vi "Perform crosstalk measurement.vi"(8 "error in (no error)":errorcluster, 10 "I2S waveforms":waveform(dbl)[](array[waveform]), 11 "measurement configuration":T2={"Full scale range"=2.825, "Channel name"="", "Analog source resource name"="", "Frequency"=0.0, "Amplitude"=0.0, "Protocol capture resource name"="", "Data line"=0, "Interferer channel"=0, "Victim channel"=0, "Sample rate"=44100.0, "Measurement duration"=0.1, "Frame sync edge for channel 0"=1, "Channel count per frame"=2, "Channel length"=32, "Bit depth"=24, "Channel 0 offset"=1, "Endiannes"=0, "Data justification"=0, "Frame length"=64, "Frame sync pulse width"=32, "Bit clock edge sync"=1}) -> (0 "error out":errorcluster, 3 "measurement results":T1)   [LabVIEW 2021, in "Crosstalk_Audio ADC.lvlib"]
uses:
  Crosstalk_Audio ADC.lvlib
  Measurement Configuration.ctl
  Measurement Results.ctl
  <vilib>/addons/_NISVFA/_Shared subVIs/Common/SVL Set dB Reference (N Ch - 1 Ref).vi
  <vilib>/addons/_NISVFA/_Spectrum Processing/SVFA Unit Conversion (Complex) (1 Ch).vi
  <vilib>/addons/_NISVFA/_Shared subVIs/Common/SVL Set dB Reference (1 Ch).vi
  <vilib>/addons/_NISVFA/_Shared subVIs/Common/svc_Log View for Spectrum (1Ch).vi
  <vilib>/addons/_NISVFA/_Spectrum Processing/SVFA Unit Conversion (1 Ch).vi
  <vilib>/addons/_NISVFA/_Shared subVIs/Common/svc_Complex Datatype Defaults.vi
  <vilib>/addons/_NISVFA/_Shared subVIs/Common/SVL Set dB Reference (variant).vi
  <vilib>/addons/_NISVFA/_Shared subVIs/Common/svc_Unwrap Phase.vi
  <vilib>/addons/_NISVFA/_Shared subVIs/Common/svc_Convert Spectrum Array to dB.vi
  <vilib>/addons/_NISVFA/_Shared subVIs/Common/svc_Spectrum Units.vi
  <vilib>/addons/_NISVFA/_Spectrum Processing/subVIs/svfa_Conversion Utility (spectrum info).vi
  <vilib>/addons/_NISVFA/_Shared subVIs/Common/svc_Format Value (DBL).vi
  <vilib>/addons/_NISVFA/_Shared subVIs/Common/svc_Get Weighting Enum and Labels.vi
  <vilib>/addons/_NISVFA/_Shared subVIs/Common/svc_Engineering Units to Unit Label.vi
  <vilib>/addons/_NISVFA/_Shared subVIs/Common/svc_Surround NonAlpha String with Parentheses.vi
  <vilib>/dlg_ctls.llb/Space Constant.vi
  <vilib>/addons/_NISVFA/_Spectrum Processing/subVIs/svfa_Peak to RMS to Peak2Peak.vi
  <vilib>/addons/_NISVFA/_Spectrum Processing/subVIs/svfa_Mag to Mag2.vi
  <vilib>/addons/_NISVFA/_Spectrum Processing/subVIs/svfa_Linear to dB.vi
  <vilib>/addons/_NISVFA/_Spectrum Processing/subVIs/svfa_dBrefA to dBrefB.vi
  <vilib>/addons/_NISVFA/_Spectrum Processing/subVIs/svfa_Spectrum to Spectral Density.vi
  <vilib>/addons/_NISVFA/_Shared subVIs/Common/svc_Unit Label Lexical Class.vi
  <vilib>/addons/_NISVFA/_Shared subVIs/Common/svc_Window Parameters.vi
  <vilib>/addons/_NISVFA/_Shared subVIs/Common/svc_Caller VI Returned in Error Source.vi
  <vilib>/addons/Sound and Vibration/svt_Single Tone Measurements/SVT Crosstalk (Time).vi
  <vilib>/Analysis/4window.llb/window parameters.vi
  <vilib>/Analysis/4window.llb/Window Properties.vi
  <vilib>/Analysis/4window.llb/Window Properties by Name.vi
  <vilib>/addons/Sound and Vibration/svt_Single Tone Measurements/SoundVib_SingleTone.lvlib
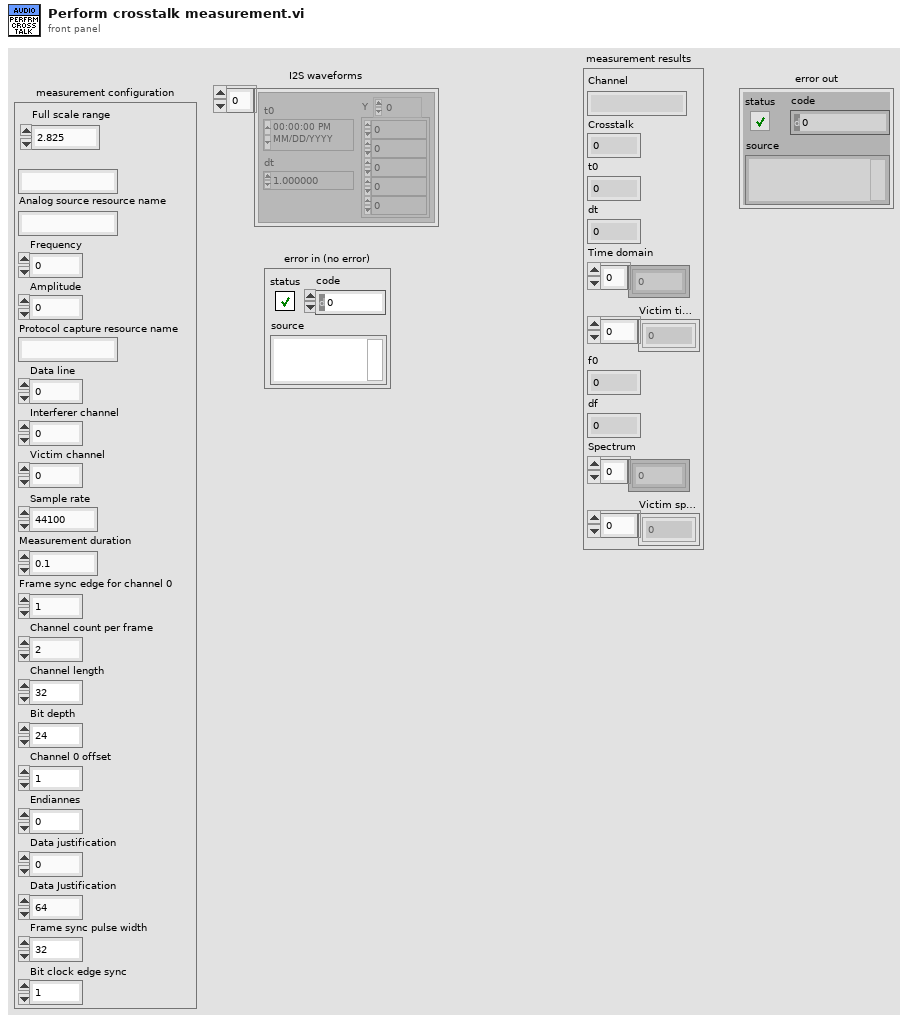
[diagram p1: front panel]
types:
  T1 = typedef "Crosstalk_Audio ADC.lvlib/Measurement Results.ctl" = cluster{"Channel":string, "Crosstalk":dbl, "t0":dbl, "dt":dbl, "Time domain":dbl[], "Victim time domain":dbl[], "f0":dbl, "df":dbl, "Spectrum":dbl[], "Victim spectrum":dbl[]}
  T2 = typedef "Crosstalk_Audio ADC.lvlib/Measurement Configuration.ctl" = cluster{"Full scale range":dbl, "Channel name":string, "Analog source resource name":string, "Frequency":dbl, "Amplitude":dbl, "Protocol capture resource name":string, "Data line":u32, "Interferer channel":u32, "Victim channel":u32, "Sample rate":dbl, "Measurement duration":dbl, "Frame sync edge for channel 0":u32, "Channel count per frame":u32, "Channel length":u32, "Bit depth":u32, "Channel 0 offset":u32, "Endiannes":u32, "Data justification":u32, "Frame length":u32, "Frame sync pulse width":u32, "Bit clock edge sync":u32}
  T3 = enum16{"no change", "spectrum", "spectral density"}
  T4 = cluster{"linear/dB":enum16{"no change", "linear", "dB"}, "dB reference (0: no change)":dbl, "power/magnitude":enum16{"no change", "power", "magnitude"}, "view":enum16{"no change", "rms", "peak", "peak-peak"}}
  T5 = typedef "svc_Spectrum Info.ctl" = cluster{"channel name":string, "description":string, "x-axis units":T6, "spectral info":cluster{"spectrum type":T7, "linear/dB":enum16{"linear", "dB"}, "window":u16, "window size":i32, "FFT size":i32}, "engineering units":T8, "custom label":string, "dB reference [EU]":dbl, "peak units":enum16{"rms", "peak", "peak-peak"}, "weighting filter":T9, "spectral density?":bool, "unit label":string, "spectrum skewed?":bool, "complimentary spectrum units":T10}
  T6 = typedef "svc_X-Axis Units.ctl" = u16
  T7 = typedef "svc_Spectrum Type.ctl" = enum16{"FFT Spectrum [complex]", "Amplitude [Magnitude]", "Power [Magnitude^2]", "Cross Spectrum [complex]", "Frequency Response [Complex]"}
  T8 = typedef "svc_Engineering Units Text Ring.ctl" = u16
  T9 = typedef "svc_Weighting Filter Text Ring.ctl" = u16
  T10 = typedef "svc_Complimentary Spectrum Units.ctl" = enum16{"none", "radians", "degrees", "cycles", "imaginary"}
  T11 = cluster{"complex spectrum response":cluster{"f0":dbl, "df":dbl, "complex spectrum":cdb[]}, "spectrum info":T5}
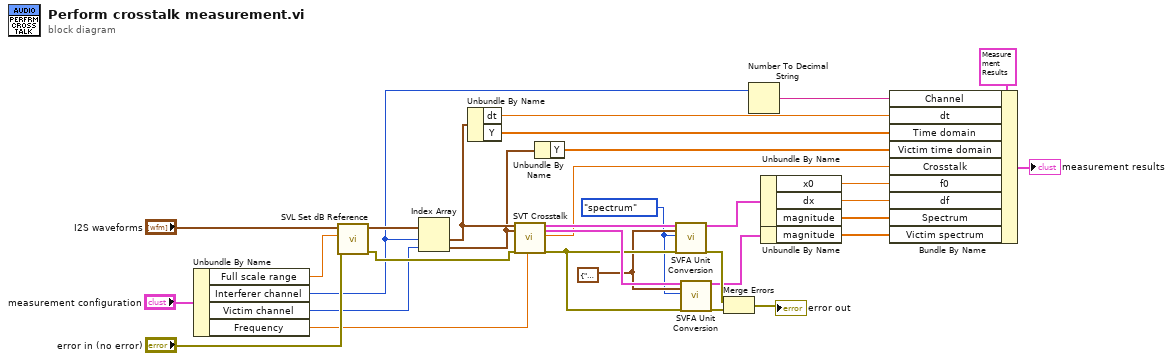
[diagram p0: block diagram]
diagram:
  w4 = T3."spectrum" ("spectral density desired")
  w5 = T4 {"linear/dB"=enum."dB", "dB reference (0: no change)"=0.0, "power/magnitude"=enum."magnitude", "view"=enum."peak-peak"} ("desired scaling")
  n1 = Unbundle By Name("measurement configuration") -> ("Full scale range"=w8:dbl, "Interferer channel"=w3:u32, "Victim channel"=w7:u32, "Frequency"=w6:dbl)
  n2 = call-poly <vilib>:"SVL Set dB Reference.vi"("error in (no error)"="error in (no error)", "dB reference [EU]"=w8, "scaled signals in [EU]"="I2S waveforms") -> ("error out"=w10:errorcluster, "scaled signals out [EU]"=w11:waveform(dbl)[])  [unwired: 7 in]
  n3 = Index Array(array=w11, index #1=w3, index #2=w7) -> (element #1=w19:waveform(dbl), element #2=w16:waveform(dbl))
  n4 = Unbundle By Name ("Get Waveform Components")(w19) -> ("dt"=w18:dbl, "Y"=w17:dbl[])
  n5 = call-poly <vilib>:"SVT Crosstalk.vi"("stimulus signal X [EUx]"=w19, "idle-channel response signal Y [EUy]"=w16, "error in (no error)"=w10, "expected fundamental frequency [Hz]"=w6) -> ("complex spectrum\nstimulus X"=w32:T11, "complex spectrum\nidle-channel response Y"=w28:T11, "crosstalk"=w20:dbl, "error out"=w27:errorcluster)  [unwired: 8 in, 4 out]
  n6 = Unbundle By Name ("Get Waveform Components")(w16) -> ("Y"=w13:dbl[])
  n7 = call-poly <vilib>:"SVFA Unit Conversion.vi"("complex spectrum"=w32, "desired scaling"=w5, "spectral density desired"=w4, "error in (no error)"=w27) -> ("converted spectrum"=w25:cluster{"x0":dbl, "dx":dbl, "magnitude":dbl[]}, "error out"=w30:errorcluster)  [unwired: 10 in, 4 out]
  n8 = call-poly <vilib>:"SVFA Unit Conversion.vi"("complex spectrum"=w28, "desired scaling"=w5, "spectral density desired"=w4, "error in (no error)"=w27) -> ("converted spectrum"=w24:cluster{"x0":dbl, "dx":dbl, "magnitude":dbl[]}, "error out"=w31:errorcluster)  [unwired: 10 in, 4 out]
  n9 = Merge Errors(w30, w31) -> (→"error out":errorcluster)
  n10 = Number To Decimal String(number=w3) -> (decimal integer string=w2:string)  [unwired: 1 in]
  n11 = Unbundle By Name(w25) -> ("x0"=w22:dbl, "dx"=w21:dbl, "magnitude"=w23:dbl[])
  n12 = Unbundle By Name(w24) -> ("magnitude"=w12:dbl[])
  n13 = Bundle By Name(cluster=T1 {"Channel"="", "Crosstalk"=0.0, "t0"=0.0, "dt"=0.0, "Time domain"=[], "Victim time domain"=[], "f0"=0.0, "df"=0.0, "Spectrum"=[], "Victim spectrum"=[]} ("measurement results"), "Channel"=w2, "dt"=w18, "Time domain"=w17, "Victim time domain"=w13, "Crosstalk"=w20, "f0"=w22, "df"=w21, "Spectrum"=w23, "Victim spectrum"=w12) -> (→"measurement results":T1)
